vi "test_Split Registers by Direction.vi"(8 "error in (no error)":errorcluster) -> (0 "error out":errorcluster)   [LabVIEW 2019, in "Load And Parse Bitfile Testing.lvclass"]
uses:
  Load And Parse Bitfile Testing.lvclass
  Addon/Addon Shared/Types/Register Information.ctl
  Addon/Addon Shared/Types/Data Type.ctl
  <vilib>/addons/_JKI Toolkits/VI Tester/TestCase.llb/TestCase.lvclass
  Addon/Addon System Explorer/FPGA Addon System Explorer.lvlib
  Addon/Addon Shared/FPGA Addon Shared.lvlib
  C:/Program Files (x86)/National Instruments/LabVIEW 2019/vi.lib/addons/_JKI Toolkits/VI Tester/TestCase.llb/TestCase.lvclass
panel:
  out "TestCase out":refnum<class "Load And Parse Bitfile Testing.lvclass">
  in  "TestCase in":refnum<class "Load And Parse Bitfile Testing.lvclass">
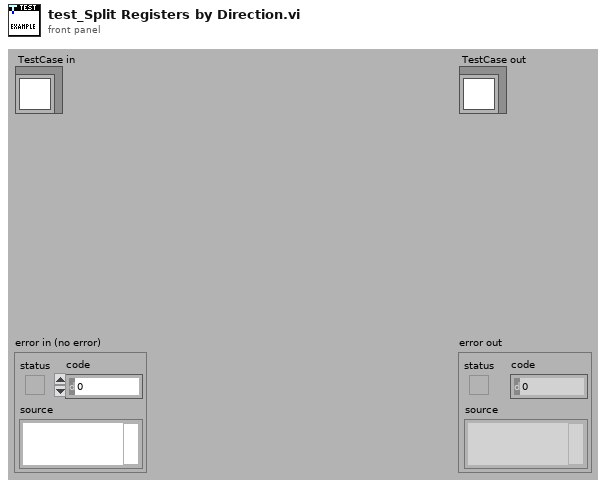
[diagram p1: front panel]
types:
  T1 = typedef "FPGA Addon Shared.lvlib/Register Information.ctl" = cluster{"Name":string, "Data Type":T2, "Default Value":variant}
  T2 = typedef "FPGA Addon Shared.lvlib/Data Type.ctl" = enum8{"<Null>", "I8", "I16", "I32", "I64", "U8", "U16", "U32", "U64", "SGL", "Boolean", "Analog PWM In Settings", "Analog PWM In", "Digital PWM In Settings", "Digital PWM In", "Digital PWM Out", "Sine Out", "FXP+/-24.5", "FXP+/-16.5", "FXP+/-32.8", "FXP+/-64.32", "FXP+/-16.7", "FXP+/-20.5", "FXP+/-27.5", "FXP+/-32.16", "FXP+16.3", "FXP+18.3", "Digital Static In", "Digital Static Out", "Digital Static In Settings", "Digital WSS Out", "Quad Encoder Settings", "Quad Encoder In", "Group"}
  T3 = typedef "niFpgaBitfileStructure_VI.ctl" = cluster{"Name":string, "RegisterMap":T4[], "Icon":T9}
  T4 = typedef "nirviControlStructure.ctl" = cluster{"Name":string, "Hidden":bool, "Indicator":bool, "Flattened Type":string, "Grouping":cluster{"Grouped":bool, "Member Names":string[], "Member IDs":u32[]}, "Address":u32, "Size":u32, "Class":u32, "Internal":bool, "Typedef":T5, "ID":u32, "Bidirectional":bool, "Synchronous":bool, "Mechanical Action":T6, "Sub Controls":T7[], "Access May Timeout":bool, "Register Node":bool}
  T5 = typedef "nirviTypdefDescription.ctl" = cluster{"Typedef":bool, "Path":path}
  T6 = typedef "nirviMechanicalAction.ctl" = enum8{"Switch When Pressed", "Switch When Released", "Switch Until Released", "Latch When Pressed", "Latch When Released", "Latch Until Released"}
  T7 = typedef "nirviSubControlStructure.ctl" = cluster{"Name":string, "flattened Type":string, "Cluster Information":T8, "Typedef":T5}
  T8 = typedef "nirviClusterElementControl.ctl" = cluster{"Name Hierarchy":string[], "Item Order":u32[]}
  T9 = typedef "imagedata.ctl" = cluster{"image type":i32, "image depth":i32, "image":u8[], "mask":u8[], "colors":u32[], "Rectangle":cluster{"left":i16, "top":i16, "right":i16, "bottom":i16}}
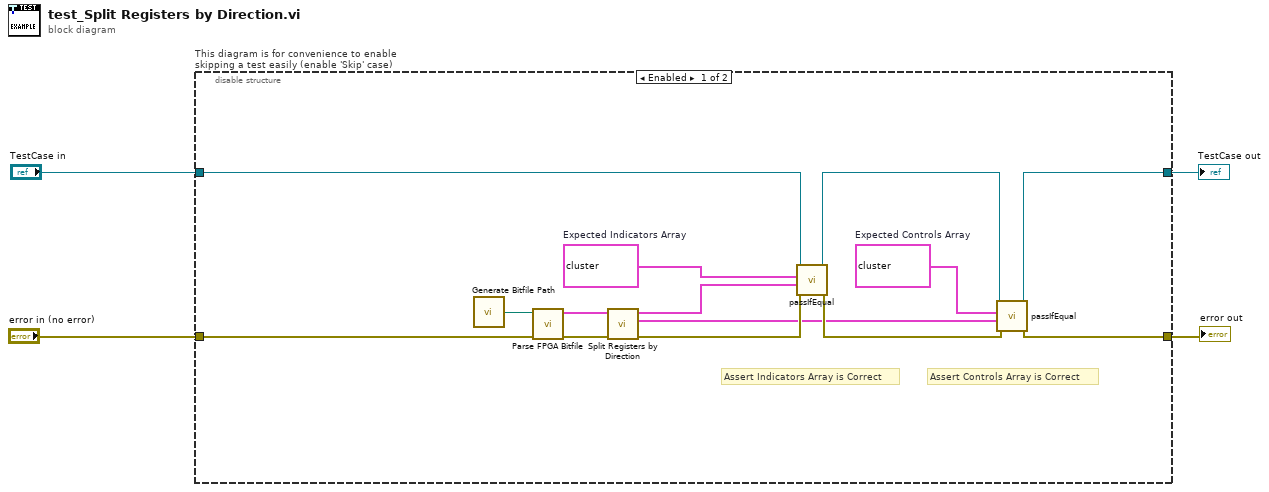
[diagram p0: block diagram]
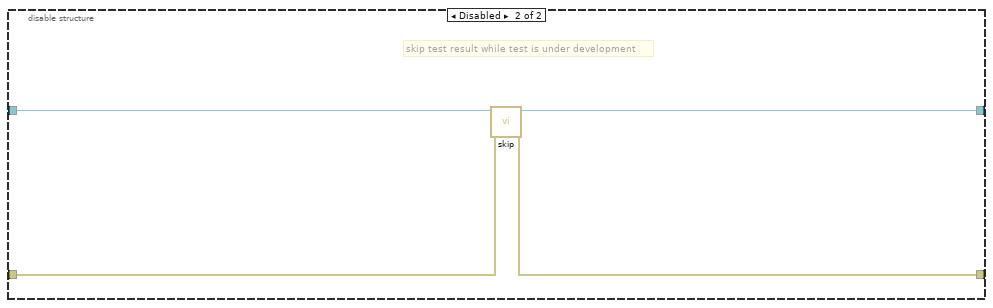
[diagram p2: hidden frame]
diagram:
  n1 = disable-structure "This diagram is for convenience to enable skipping a test easily (enable 'Skip' case)" shown="Enabled" {
    disable-tunnel: "TestCase in" -> [w18 w22]
    disable-tunnel: [w8 w20] -> w1
    disable-tunnel: [w12 w21] -> w3
    disable-tunnel: "error in (no error)" -> [w17 w19]
    frame Enabled {
      w6 = T1[] [{"Name"="Boolean", "Data Type"=enum."Boolean", "Default Value"=variant(dbl 0.0)}, {"Name"="FXP16.3", "Data Type"=enum."FXP+16.3", "Default Value"=variant(fxp<+,16,3> 0.0)}, {"Name"="FXP16.5", "Data Type"=enum."FXP+/-16.5", "Default Value"=variant(fxp<+/-,16,5> 0.0)}, {"Name"="FXP16.7", "Data Type"=enum."FXP+/-16.7", "Default Value"=variant(fxp<+/-,16,7> 0.0)}, {"Name"="FXP18.3", "Data Type"=enum."FXP+18.3", "Default Value"=variant(fxp<+,18,3> 0.0)}, {"Name"="FXP20.5", "Data Type"=enum."FXP+/-20.5", "Default Value"=variant(fxp<+/-,20,5> 0.0)}, {"Name"="FXP24.5", "Data Type"=enum."FXP+/-24.5", "Default Value"=variant(fxp<+/-,24,5> 0.0)}, {"Name"="FXP27.5", "Data Type"=enum."FXP+/-27.5", "Default Value"=variant(fxp<+/-,27,5> 0.0)}, {"Name"="FXP32.16", "Data Type"=enum."FXP+/-32.16", "Default Value"=variant(fxp<+/-,32,16> 0.0)}, {"Name"="FXP32.8", "Data Type"=enum."FXP+/-32.8", "Default Value"=variant(fxp<+/-,32,8> 0.0)}, {"Name"="FXP64.32", "Data Type"=enum."FXP+/-64.32", "Default Value"=variant(fxp<+/-,64,32> 0.0)}, {"Name"="Group1.I16", "Data Type"=enum."I16", "Default Value"=variant(dbl 0.0)}, {"Name"="Group1.I32", "Data Type"=enum."I32", "Default Value"=variant(dbl 0.0)}, {"Name"="Group1.I64", "Data Type"=enum."I64", "Default Value"=variant(dbl 0.0)}, {"Name"="Group1.I8", "Data Type"=enum."I8", "Default Value"=variant(dbl 0.0)}, {"Name"="Group1.SGL", "Data Type"=enum."SGL", "Default Value"=variant(dbl 0.0)}, {"Name"="Group1.U16", "Data Type"=enum."U16", "Default Value"=variant(dbl 0.0)}, {"Name"="Group1.U32", "Data Type"=enum."U32", "Default Value"=variant(dbl 0.0)}, {"Name"="Group1.U64", "Data Type"=enum."U64", "Default Value"=variant(dbl 0.0)}, {"Name"="Group1.U8", "Data Type"=enum."U8", "Default Value"=variant(dbl 0.0)}, {"Name"="Group2.Boolean", "Data Type"=enum."Boolean", "Default Value"=variant(dbl 0.0)}, {"Name"="Group2.FXP16.3", "Data Type"=enum."FXP+16.3", "Default Value"=variant(fxp<+,16,3> 0.0)}, {"Name"="Group2.FXP16.5", "Data Type"=enum."FXP+/-16.5", "Default Value"=variant(fxp<+/-,16,5> 0.0)}, {"Name"="Group2.FXP16.7", "Data Type"=enum."FXP+/-16.7", "Default Value"=variant(fxp<+/-,16,7> 0.0)}, {"Name"="Group2.FXP18.3", "Data Type"=enum."FXP+18.3", "Default Value"=variant(fxp<+,18,3> 0.0)}, {"Name"="Group2.FXP20.5", "Data Type"=enum."FXP+/-20.5", "Default Value"=variant(fxp<+/-,20,5> 0.0)}, {"Name"="Group2.FXP24.5", "Data Type"=enum."FXP+/-24.5", "Default Value"=variant(fxp<+/-,24,5> 0.0)}, {"Name"="Group2.FXP27.5", "Data Type"=enum."FXP+/-27.5", "Default Value"=variant(fxp<+/-,27,5> 0.0)}, {"Name"="Group2.FXP32.16", "Data Type"=enum."FXP+/-32.16", "Default Value"=variant(fxp<+/-,32,16> 0.0)}, {"Name"="Group2.FXP32.8", "Data Type"=enum."FXP+/-32.8", "Default Value"=variant(fxp<+/-,32,8> 0.0)}, {"Name"="Group2.FXP64.32", "Data Type"=enum."FXP+/-64.32", "Default Value"=variant(fxp<+/-,64,32> 0.0)}, {"Name"="I16", "Data Type"=enum."I16", "Default Value"=variant(dbl 0.0)}, {"Name"="I32", "Data Type"=enum."I32", "Default Value"=variant(dbl 0.0)}, {"Name"="I64", "Data Type"=enum."I64", "Default Value"=variant(dbl 0.0)}, {"Name"="I8", "Data Type"=enum."I8", "Default Value"=variant(dbl 0.0)}, {"Name"="SGL", "Data Type"=enum."SGL", "Default Value"=variant(dbl 0.0)}, {"Name"="U16", "Data Type"=enum."U16", "Default Value"=variant(dbl 0.0)}, {"Name"="U32", "Data Type"=enum."U32", "Default Value"=variant(dbl 0.0)}, {"Name"="U64", "Data Type"=enum."U64", "Default Value"=variant(dbl 0.0)}, {"Name"="U8", "Data Type"=enum."U8", "Default Value"=variant(dbl 0.0)}]  # Expected Controls Array
      w7 = T1[] [{"Name"="Boolean out", "Data Type"=enum."Boolean", "Default Value"=variant(dbl 0.0)}, {"Name"="FXP16.3 out", "Data Type"=enum."FXP+16.3", "Default Value"=variant(fxp<+,16,3> 0.0)}, {"Name"="FXP16.5 out", "Data Type"=enum."FXP+/-16.5", "Default Value"=variant(fxp<+/-,16,5> 0.0)}, {"Name"="FXP16.7 out", "Data Type"=enum."FXP+/-16.7", "Default Value"=variant(fxp<+/-,16,7> 0.0)}, {"Name"="FXP18.3 out", "Data Type"=enum."FXP+18.3", "Default Value"=variant(fxp<+,18,3> 0.0)}, {"Name"="FXP20.5 out", "Data Type"=enum."FXP+/-20.5", "Default Value"=variant(fxp<+/-,20,5> 0.0)}, {"Name"="FXP24.5 out", "Data Type"=enum."FXP+/-24.5", "Default Value"=variant(fxp<+/-,24,5> 0.0)}, {"Name"="FXP27.5 out", "Data Type"=enum."FXP+/-27.5", "Default Value"=variant(fxp<+/-,27,5> 0.0)}, {"Name"="FXP32.16 out", "Data Type"=enum."FXP+/-32.16", "Default Value"=variant(fxp<+/-,32,16> 0.0)}, {"Name"="FXP32.8 out", "Data Type"=enum."FXP+/-32.8", "Default Value"=variant(fxp<+/-,32,8> 0.0)}, {"Name"="FXP64.32 out", "Data Type"=enum."FXP+/-64.32", "Default Value"=variant(fxp<+/-,64,32> 0.0)}, {"Name"="Fast timeout", "Data Type"=enum."Boolean", "Default Value"=variant(dbl 0.0)}, {"Name"="Fast timeout 2", "Data Type"=enum."Boolean", "Default Value"=variant(dbl 0.0)}, {"Name"="Fast timeout 3", "Data Type"=enum."Boolean", "Default Value"=variant(dbl 0.0)}, {"Name"="Group1.I16 out", "Data Type"=enum."I16", "Default Value"=variant(dbl 0.0)}, {"Name"="Group1.I32 out", "Data Type"=enum."I32", "Default Value"=variant(dbl 0.0)}, {"Name"="Group1.I64 out", "Data Type"=enum."I64", "Default Value"=variant(dbl 0.0)}, {"Name"="Group1.I8 out", "Data Type"=enum."I8", "Default Value"=variant(dbl 0.0)}, {"Name"="Group1.SGL out", "Data Type"=enum."SGL", "Default Value"=variant(dbl 0.0)}, {"Name"="Group1.U16 out", "Data Type"=enum."U16", "Default Value"=variant(dbl 0.0)}, {"Name"="Group1.U32 out", "Data Type"=enum."U32", "Default Value"=variant(dbl 0.0)}, {"Name"="Group1.U64 out", "Data Type"=enum."U64", "Default Value"=variant(dbl 0.0)}, {"Name"="Group1.U8 out", "Data Type"=enum."U8", "Default Value"=variant(dbl 0.0)}, {"Name"="Group2.Boolean out", "Data Type"=enum."Boolean", "Default Value"=variant(dbl 0.0)}, {"Name"="Group2.FXP16.3 out", "Data Type"=enum."FXP+16.3", "Default Value"=variant(fxp<+,16,3> 0.0)}, {"Name"="Group2.FXP16.5 out", "Data Type"=enum."FXP+/-16.5", "Default Value"=variant(fxp<+/-,16,5> 0.0)}, {"Name"="Group2.FXP16.7 out", "Data Type"=enum."FXP+/-16.7", "Default Value"=variant(fxp<+/-,16,7> 0.0)}, {"Name"="Group2.FXP18.3 out", "Data Type"=enum."FXP+18.3", "Default Value"=variant(fxp<+,18,3> 0.0)}, {"Name"="Group2.FXP20.5 out", "Data Type"=enum."FXP+/-20.5", "Default Value"=variant(fxp<+/-,20,5> 0.0)}, {"Name"="Group2.FXP24.5 out", "Data Type"=enum."FXP+/-24.5", "Default Value"=variant(fxp<+/-,24,5> 0.0)}, {"Name"="Group2.FXP27.5 out", "Data Type"=enum."FXP+/-27.5", "Default Value"=variant(fxp<+/-,27,5> 0.0)}, {"Name"="Group2.FXP32.16 out", "Data Type"=enum."FXP+/-32.16", "Default Value"=variant(fxp<+/-,32,16> 0.0)}, {"Name"="Group2.FXP32.8 out", "Data Type"=enum."FXP+/-32.8", "Default Value"=variant(fxp<+/-,32,8> 0.0)}, {"Name"="Group2.FXP64.32 out", "Data Type"=enum."FXP+/-64.32", "Default Value"=variant(fxp<+/-,64,32> 0.0)}, {"Name"="I16 out", "Data Type"=enum."I16", "Default Value"=variant(dbl 0.0)}, {"Name"="I32 out", "Data Type"=enum."I32", "Default Value"=variant(dbl 0.0)}, {"Name"="I64 out", "Data Type"=enum."I64", "Default Value"=variant(dbl 0.0)}, {"Name"="I8 out", "Data Type"=enum."I8", "Default Value"=variant(dbl 0.0)}, {"Name"="Med timeout", "Data Type"=enum."Boolean", "Default Value"=variant(dbl 0.0)}, {"Name"="SGL out", "Data Type"=enum."SGL", "Default Value"=variant(dbl 0.0)}, {"Name"="Slow timeout", "Data Type"=enum."Boolean", "Default Value"=variant(dbl 0.0)}, {"Name"="U16 out", "Data Type"=enum."U16", "Default Value"=variant(dbl 0.0)}, {"Name"="U32 out", "Data Type"=enum."U32", "Default Value"=variant(dbl 0.0)}, {"Name"="U64 out", "Data Type"=enum."U64", "Default Value"=variant(dbl 0.0)}, {"Name"="U8 out", "Data Type"=enum."U8", "Default Value"=variant(dbl 0.0)}]  # Expected Indicators Array
      # "Assert Controls Array is Correct"
      # "Assert Indicators Array is Correct"
      n2 = call "Generate Bitfile Path.vi"() -> ("Bitfile Path"=w5:path)
      n3 = call "Parse FPGA Bitfile.vi"("error in (no error)"=w17, "Path"=w5) -> ("error out"=w16:errorcluster, "vi info"=w15:T3)  [unwired: 7 in, 1 out]
      n4 = call "Split Registers by Direction.vi"("error in"=w16, "vi info"=w15) -> ("error out"=w14:errorcluster, "Controls"=w10:T1[], "Indicator"=w13:T1[])  [unwired: 7 in]
      n5 = call-dynamic "passIfEqual.vi"("error in (no error)"=w14, "y"=w13, "x"=w7, "TestCase in"=w18) -> ("error out"=w11:errorcluster, "TestCase out"=w9:refnum<class "Load And Parse Bitfile Testing.lvclass">)  [unwired: 6 in]
      n6 = call-dynamic "passIfEqual.vi"("error in (no error)"=w11, "y"=w10, "x"=w6, "TestCase in"=w9) -> ("error out"=w12:errorcluster, "TestCase out"=w8:refnum<class "Load And Parse Bitfile Testing.lvclass">)  [unwired: 6 in]
    }
    frame Disabled {
      # "skip test result while test is under development"
      n7 = call <vilib>:"skip.vi"("error in (no error)"=w19, "TestCase in"=w22) -> ("error out"=w21:errorcluster, "TestCase out"=w20:refnum<class "Load And Parse Bitfile Testing.lvclass">)  [unwired: 8 in]
    }
  }
  "error out" <- w3
  "TestCase out" <- w1
